vi "1.2.vi"(8 "error in (no error)":errorcluster, 10 "input":string) -> (0 "error out":errorcluster, 2 "Out":dbl)   [LabVIEW 2017]
panel:
  out "Array":dbl[](array[numeric])
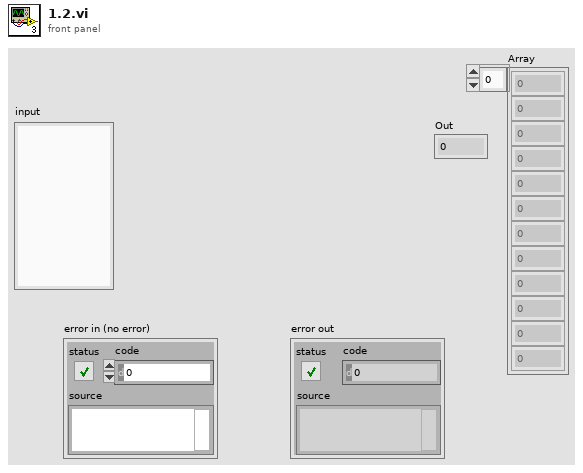
[diagram p1: front panel]
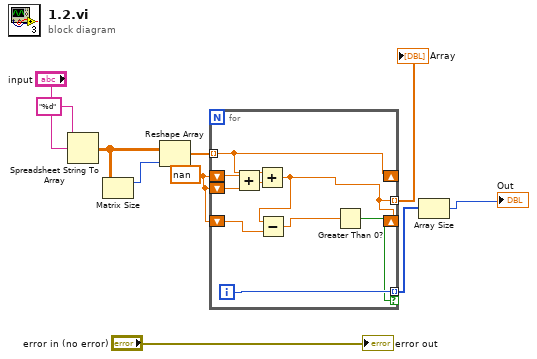
[diagram p0: block diagram]
diagram:
  w1 = nan
  n1 = Spreadsheet String To Array(format string="%d" ("delimiter (Tab)"), spreadsheet string="input") -> (array=w7:dbl[][])  [unwired: 2 in]
  n2 = Matrix Size(0:w7) -> (1:w6:i32)  [unwired: 1 out]
  n3 = Reshape Array(w7, w6) -> (w5:dbl[])
  n4 = for {
    tunnel: w5 -> [w14] mode=indexing
    shift-right: [w14] -> _
    shift-left: w1 -> [w16]
    tunnel: [w19] -> w4 mode=indexing if=w18
    shift-left: w1 -> [w17]
    tunnel: [w13] -> w2 mode=indexing
    shift-right: [w13] -> _
    shift-left: w1 -> [w12]
    i -> [w19]
    n5 = Add(x=w16, y=w17) -> (x+y=w15:dbl)
    n6 = Add(x=w14, y=w15) -> (x+y=w13:dbl)
    n7 = Subtract(x=w13, y=w12) -> (x-y=w11:dbl)
    n8 = Greater Than 0?(x=w11) -> (x > 0?=w18:bool)
  }
  "Array" <- w2
  n9 = Array Size(array=w4) -> (size(s)=→"Out":i32)
  "error out" <- "error in (no error)"
